vi "Export Custom Device Configuration.vi"(6 "operation":T1(ring)=enum."replace or create with confirmation", 8 "error in (no error)":errorcluster, 9 "File Interface in":refnum<class "File Interface.lvclass">, 10 "Path":path, 11 "ID":u64) -> (0 "error out":errorcluster, 3 "ID out":u64)   [LabVIEW 2027, in "ImportExport.lvlib"]
doc: "ExportCDConfig.vi saves a configuration file (.dat) that can be later loaded using ImportCDConfig.vi. This configuration file includes the values for the properties of each Section, Channel, or Waveform in your Custom Device. You can add this functionality as a Button, Runtime Menu, or as a property for one of your Channels."
uses:
  ImportExport.lvlib
  File Interface Class/File Interface.lvclass
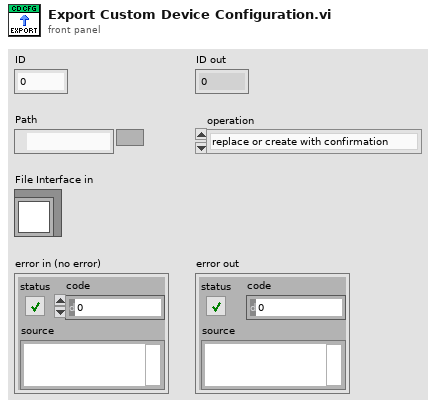
[diagram p1: front panel]
types:
  T1 = enum16{"open", "replace", "create", "open or create", "replace or create", "replace or create with confirmation"}
  T2 = typedef "Advanced System Definition.lvlib/SysDef.Export.ctl" = cluster{"Version":string, "Tree":T3[]}
  T3 = typedef "Advanced System Definition.lvlib/TreeItem.ctl" = cluster{"Item Info":T4, "Parent Path":string[], "Properties":T9[]}
  T4 = typedef "Advanced System Definition.lvlib/TreeItem.Info.ctl" = cluster{"Name":string, "Description":string, "GUID":string, "Is Channel":bool, "Channel":T5, "Is Waveform":bool, "Waveform":T7}
  T5 = typedef "Custom Device API.lvlib/Custom Device Channel.ctl" = cluster{"Type":T6, "Units":string, "Default Value":dbl, "Faultable":bool, "Scalable":bool}
  T6 = typedef "Custom Device API.lvlib/Custom Device Channel Type.ctl" = enum16{"Input", "Output"}
  T7 = typedef "Custom Device API.lvlib/Custom Device Waveform.ctl" = cluster{"Data Type":T8, "Units":string}
  T8 = typedef "Custom Device API.lvlib/Custom Device Waveform DataType.ctl" = enum16{"Double", "Complex Double"}
  T9 = typedef "Advanced System Definition.lvlib/TreeItem.Property.ctl" = cluster{"Name":string, "Type":i32, "Value":variant}
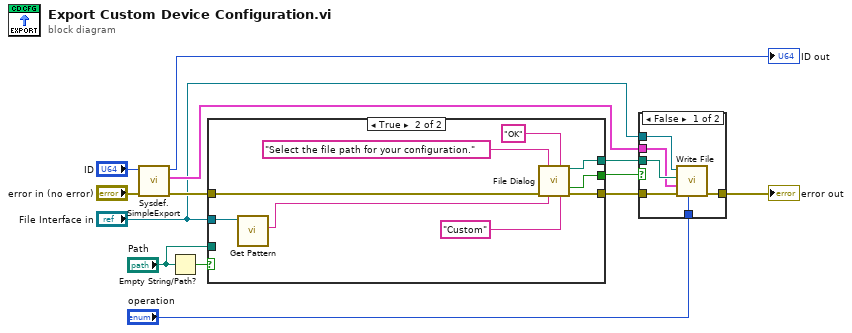
[diagram p0: block diagram]
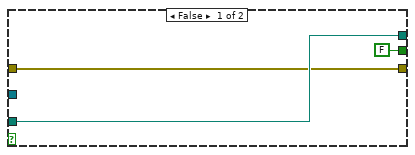
[diagram p2: hidden frame]
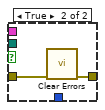
[diagram p3: hidden frame]
diagram:
  n1 = call "Sysdef.SimpleExport.vi"("error in (no error)"="error in (no error)", "ID"="ID") -> ("error out"=w13:errorcluster, "Export"=w12:T2, "ID out"=→"ID out":u64)  [unwired: 7 in]
  n2 = Empty String/Path?(string/path="Path") -> (empty?=w4:bool)
  n3 = case shown="True" w4 {
    tunnel: w13 -> [w15 w25]
    tunnel: "File Interface in" -> [_ w24]
    tunnel: [FALSE ("cancelled") w20] -> w7
    tunnel: [w15 w19] -> w6
    tunnel: [w16 w18] -> w5
    tunnel: "Path" -> [w16 _]
    frame False {
    }
    frame True {
      n4 = call-dynamic "Get Pattern.vi"("File Interface in"=w24) -> ("file extension"=w17:string)  [unwired: 10 in]
      n5 = call "File Dialog"("prompt"="Select the file path for your configuration.", "button label"="OK", "error in"=w25, "pattern (all files)"=w17, "pattern label"="Custom") -> ("selected path"=w18:path, "cancelled"=w20:bool, "error out"=w19:errorcluster)  [unwired: 7 in, 1 out]
    }
  }
  n6 = case shown="False" w7 {
    tunnel: [w27 w32] -> w8
    tunnel: w6 -> [w28 w33]
    tunnel: w5 -> [w30 _]
    tunnel: w12 -> [w29 _]
    tunnel: "File Interface in" -> [w31 _]
    tunnel: "operation" -> [w26 _]
    frame False {
      n7 = call-dynamic "Write File.vi"("operation"=w26, "error in (no error)"=w28, "Data"=w29, "datalog path (use dialog)"=w30, "File Interface in"=w31) -> ("error out"=w27:errorcluster)  [unwired: 6 in]
    }
    frame True {
      n8 = call <vilib>:"Clear Errors.vi"("error in (no error)"=w33) -> ("error out"=w32:errorcluster)  [unwired: 5 in, 1 out]
    }
  }
  "error out" <- w8
